vi "TestPMUData.vi"() -> ()   [LabVIEW 2018]
uses:
  SensorShared/clSensorData.ctl
  C37.118 PMU.lvclass
  <userlib>/NIST/Socket Class/Classes/Socket.Base/Socket.Base.lvclass
  SensorShared/SensorShared.lvlib
panel:
  out "clSensorData":T1
  out "error out":errorcluster
  in  "stop":bool
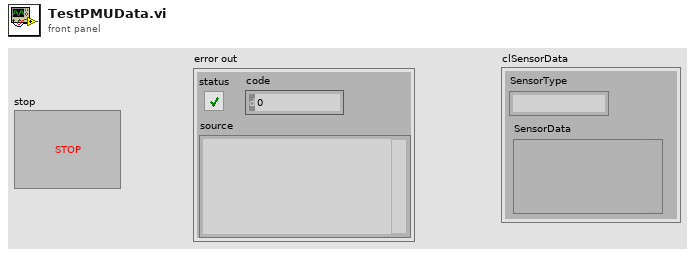
[diagram p1: front panel]
types:
  T1 = typedef "SensorShared.lvlib/clSensorData.ctl" = cluster{"SensorType":string, "SensorData":variant}
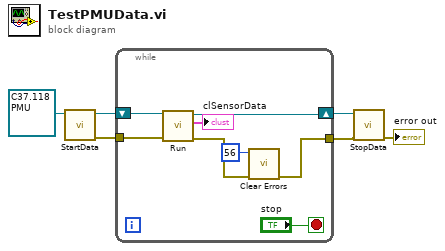
[diagram p0: block diagram]
diagram:
  n1 = call-dynamic "StartData.vi"("Class In"=refnum<class "C37.118 PMU.lvclass"> refnum) -> ("error out"=w4:errorcluster, "Class Out"=w5:refnum<class "C37.118 PMU.lvclass">)  [unwired: 9 in]
  n2 = while {
    shift-right: [w11] -> w2
    shift-left: w5 -> [w13]
    tunnel: w4 -> [w12]
    tunnel: [w9] -> w3
    stop <- "stop" stop-if-true
    n3 = call-dynamic "Run.vi"("error in (no error)"=w12, "C37.118 PMU in"=w13) -> ("error out"=w10:errorcluster, "clSensorData"=→"clSensorData":T1, "C37.118 PMU out"=w11:refnum<class "C37.118 PMU.lvclass">)  [unwired: 6 in, 1 out]
    n4 = call <vilib>:"Clear Errors.vi"("error in (no error)"=w10, "specific error code to clear (0: all)"=56) -> ("error out"=w9:errorcluster)  [unwired: 4 in, 1 out]
  }
  n5 = call-dynamic "StopData.vi"("error in (no error)"=w3, "Class In"=w2) -> ("error out"=→"error out":errorcluster)  [unwired: 8 in, 1 out]
